vi "Read size.vi"(11 "ITem in":refnum<class "file_Item.lvclass">) -> (3 "size":u32)   [LabVIEW 2020, in "file_Item.lvclass"]
uses:
  file_Item.lvclass
  file_Item.lvclass/file_Item.ctl
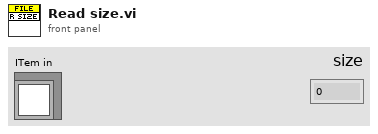
[diagram p1: front panel]
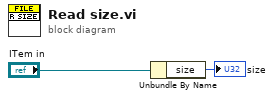
[diagram p0: block diagram]
diagram:
  n1 = Unbundle By Name("ITem in") -> ("size"=→"size":u32)
